vi "Drive Controller.vi"(8 "error in":errorcluster) -> ()   [LabVIEW 2017]
doc: "This VI executes continuously carrying out the current operation and responding to updates or new operation requests. It will often contain the timing or control code that is difficult to place directly in TeleOp. This VI generally opens all sensors and motors and isolates the rest of the robot code from knowing implementation details of how the operations are carried out."
uses:
  Drive Setpoints.ctl
  Drive Operations.ctl
  <vilib>/Rock Robotics/WPI/Solenoid/WPI_SolenoidChannel.ctl
  <vilib>/Rock Robotics/WPI/SafetyOutput/WPI_SafetyOutputConfigMenu.ctl
  Users/Public/Documents/Cross The Road Electronics/Phoenix-LabVIEW/Motor Controller/Controls/CTRE_Phoenix_MotorControl_ControlMode.ctl
  <vilib>/Rock Robotics/WPI/ThirdParty/Phoenix-LabVIEW/Motor Controller/Controls/CTRE_Phoenix_MotorControl_NeutralMode.ctl
  <vilib>/Rock Robotics/WPI/ThirdParty/Phoenix-LabVIEW/Motor Controller/Controls/CTRE_Phoenix_MotorControl_FeedbackDevice.ctl
  <vilib>/Rock Robotics/WPI/Solenoid/WPI_SolenoidValue.ctl
  <vilib>/Rock Robotics/WPI/ThirdParty/Phoenix-LabVIEW/Motor Controller/Controls/CTRE_Phoenix_MotorControl_StatusFrameEnhanced.ctl
  <vilib>/Rock Robotics/WPI/Solenoid/WPI_SolenoidOpenSingle.vi
  <vilib>/Rock Robotics/WPI/Solenoid/WPI_SolenoidSetEnum.vi
  <vilib>/Rock Robotics/WPI/Utilities/WPI_GetSetVariantRefNum.vi
  <vilib>/Rock Robotics/WPI/RobotDrive/WPI_RobotDriveMecanumDrive_Cartesian.vi
  <vilib>/Rock Robotics/WPI/ThirdParty/Phoenix-LabVIEW/Motor Controller/Get/CTRE_Phoenix_MotorController_GetQuadratureData.vi
panel:
  in  "P 2":dbl=0.8 format="%#_13g"
  in  "D":dbl format="%#_13g"
  in  "F 2":dbl=0.578
  in  "F":dbl=0.578
  out "Current\nCmd":string
  # ".578"
  # "Tip: It may be helpful to observe inputs and sensor values.\nYou may also want to display tuning or debugging controls."
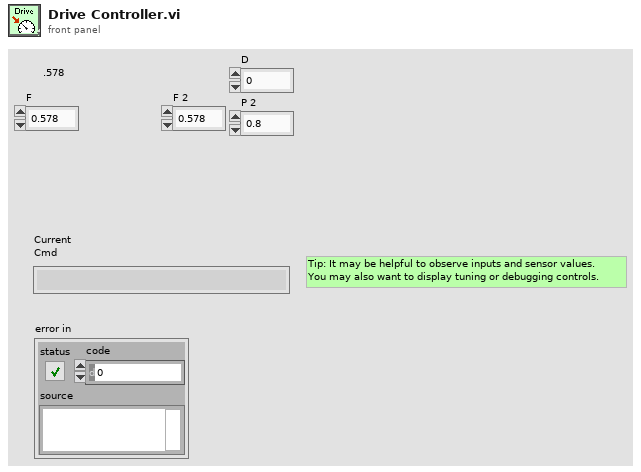
[diagram p1: front panel]
types:
  T1 = typedef "WPI_SolenoidChannel.ctl" = enum8{"Solenoid 0", "Solenoid 1", "Solenoid 2", "Solenoid 3", "Solenoid 4", "Solenoid 5", "Solenoid 6", "Solenoid 7", "Invalid"}
  T2 = typedef "CTRE_Phoenix_MotorControl_FeedbackDevice.ctl" = i8
  T3 = typedef "CTRE_Phoenix_MotorControl_NeutralMode.ctl" = enum8{"EEPROMSetting", "Override to Coast", "Override to Brake"}
  T4 = typedef "CTRE_Phoenix_MotorControl_ControlMode.ctl" = u16
  T5 = typedef "WPI_SafetyOutputConfigMenu.ctl" = enum16{"Enable", "Disable"}
  T6 = typedef "Drive Setpoints.ctl" = cluster{"Operation":T7, "X Setpoint":dbl, "Y Setpoint":dbl, "Duration":dbl, "Z Setpoint":dbl, "Tracks":bool, "Gyro":dbl, "POV":i16, "Distance(feet)":dbl, "AutoTrack Toggle":bool, "Collsision Detection":bool, "Reset Encoder":bool, "MP File Name":string}
  T7 = typedef "Drive Operations.ctl" = enum16{"Reserve", "Read Current", "Reset Motors VBus", "Motion Profile run", "Immediate Robot Centric", "Drive for Time Robot Centric", "Immediate Field Centric", "Drive For Time Field Centric", "Button Adjust", "Set Motors Motion Profile", "Reset Encoders", "Motion Profile Enable", "Drive for Distance"}
  T8 = typedef "WPI_MotorControlDeviceRef.ctl" = cluster{"DeviceStatus":errorcluster, "Type":T9, "PWM":cluster{"PWM Channel":T10, "DeadBand":T11}, "CAN":cluster{"Device Number":u8, "SetOutput VI Ref":variant, "GetOutput VI Ref":variant, "Enable VI Ref":variant, "Disable VI Ref":variant, "Data":variant}, "Invert":bool, "DIO PWM":cluster{"PWM \"Enable\" Channel":T10, "DIOChannel":T12, "PWM Rate":dbl}}
  T9 = typedef "WPI_MotorControlType.ctl" = enum16{"PWM", "CAN", "DIO PWM"}
  T10 = typedef "FPGA_DIOPWMChannel.ctl" = enum8{"PWM 0", "PWM 1", "PWM 2", "PWM 3", "PWM 4", "PWM 5", "PWM 6", "PWM 7", "PWM 8", "PWM 9", "PWM MXP 0", "PWM MXP 1", "PWM MXP 2", "PWM MXP 3", "PWM MXP 4", "PWM MXP 5", "PWM MXP 6", "PWM MXP 7", "PWM MXP 8", "PWM MXP 9", "Invalid"}
  T11 = typedef "WPI_PWMDeadband.ctl" = cluster{"Name":string, "maxPositivePwm":i32, "minPositivePwm":i32, "centerPwm":i32, "maxNegativePwm":i32, "minNegativePwm":i32, "angularRange":u16}
  T12 = typedef "FPGA_DIOChannel.ctl" = enum8{"DIO 0", "DIO 1", "DIO 2", "DIO 3", "DIO 4", "DIO 5", "DIO 6", "DIO 7", "DIO 8", "DIO 9", "DIO MXP 0", "DIO MXP 1", "DIO MXP 2", "DIO MXP 3", "DIO MXP 4", "DIO MXP 5", "DIO MXP 6", "DIO MXP 7", "DIO MXP 8", "DIO MXP 9", "DIO MXP 10", "DIO MXP 11", "DIO MXP 12", "DIO MXP 13", "DIO MXP 14", "DIO MXP 15", "SPI Port CS1", "SPI Port CS2", "SPI Port CS3", "SPI Port MISO", "SPI Port MOSI", "Invalid"}
  T13 = typedef "WPI_RobotDriveDevRef.ctl" = cluster{"DevStatus":errorcluster, "Motors[]":T8[], "Square Inputs":bool, "Max Output":dbl}
  T14 = typedef "WPI_SolenoidDevRef.ctl" = cluster{"DevStatus":errorcluster, "Pneumatics Control Module":u8, "Forward Solenoid Channel":T1, "Reverse Solenoid Channel":T1}
  T15 = typedef "Command Status Info.ctl" = cluster{"Name":string, "Status":T16, "notifier out":T17}
  T16 = typedef "Completion Status.ctl" = enum16{"Successful", "Aborted", "Incomplete"}
  T17 = typedef "Completion Notifier.ctl" = refnum<notifier>
  T18 = cluster{"SubSystem Data":T6, cluster{"Start Time (ms)":u32, "Iterations":i32}, cluster{"Command Info":T15, "Description":string, "SubSystem Data":T6, "notifier out":refnum<notifier>, "Subsystem Name":string}}
  T19 = typedef "WPI_SolenoidValue.ctl" = enum16{"Off", "On", "Forward", "Reverse"}
  T20 = typedef "CTRE_Phoenix_MotorControl_StatusFrameEnhanced.ctl" = u16
  T21 = cluster{"SubSystem Data":T6, cluster{"Start Time (ms)":u32, "Iterations":i32}, "Default Command Arguments":cluster{"Command Info":T15, "Description":string, "SubSystem Data":T6, "notifier out":refnum<notifier>, "Subsystem Name":string}}
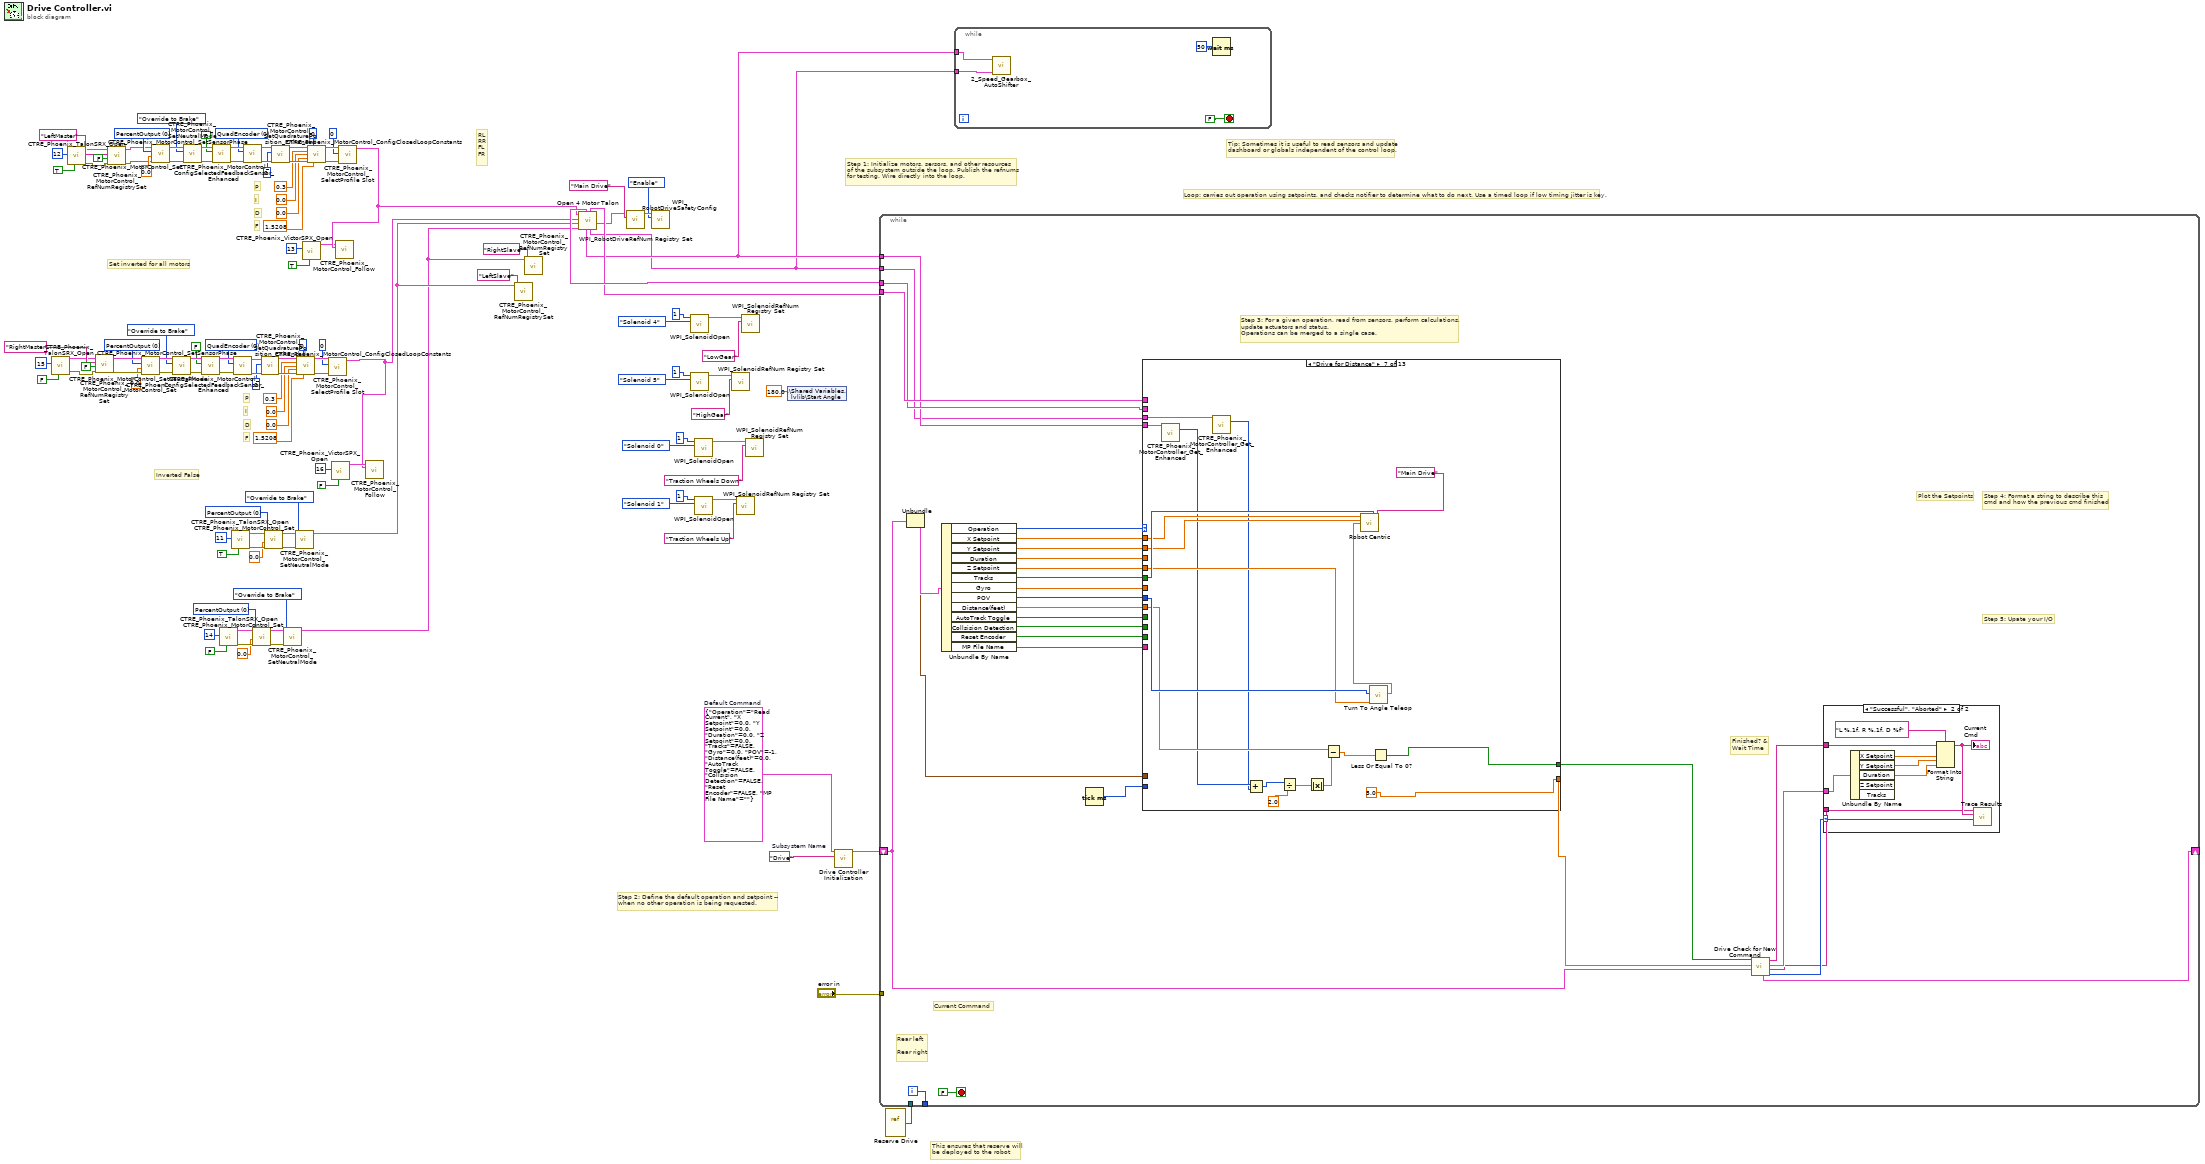
[diagram p0: block diagram]
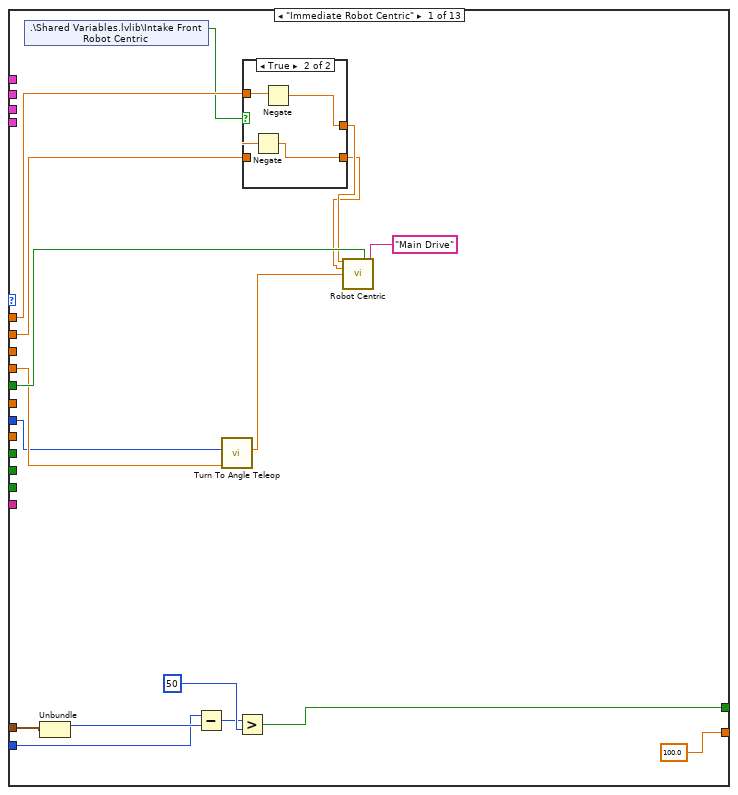
[diagram p3: hidden frame]
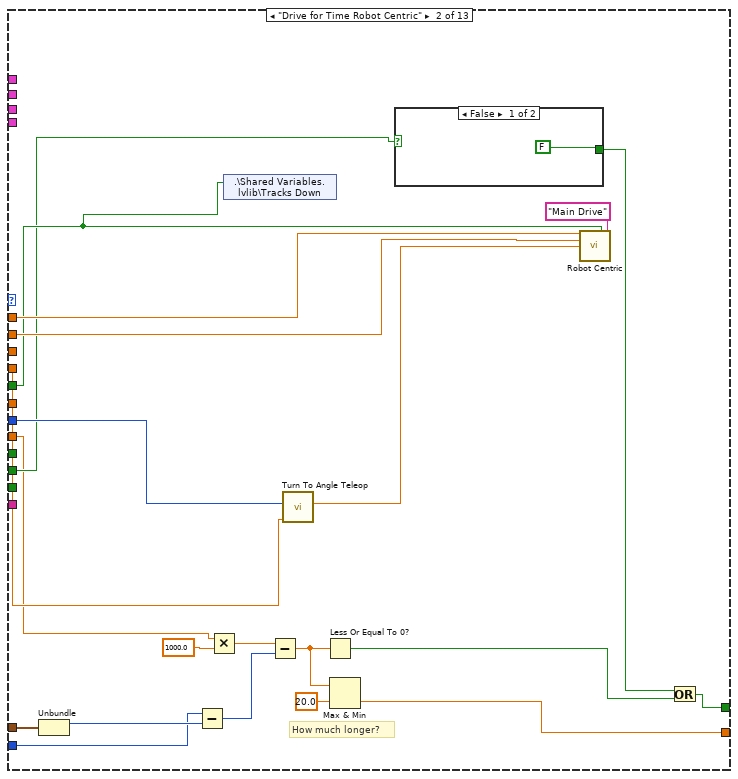
[diagram p5: hidden frame]
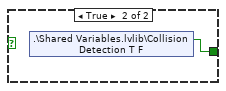
[diagram p6: hidden frame]
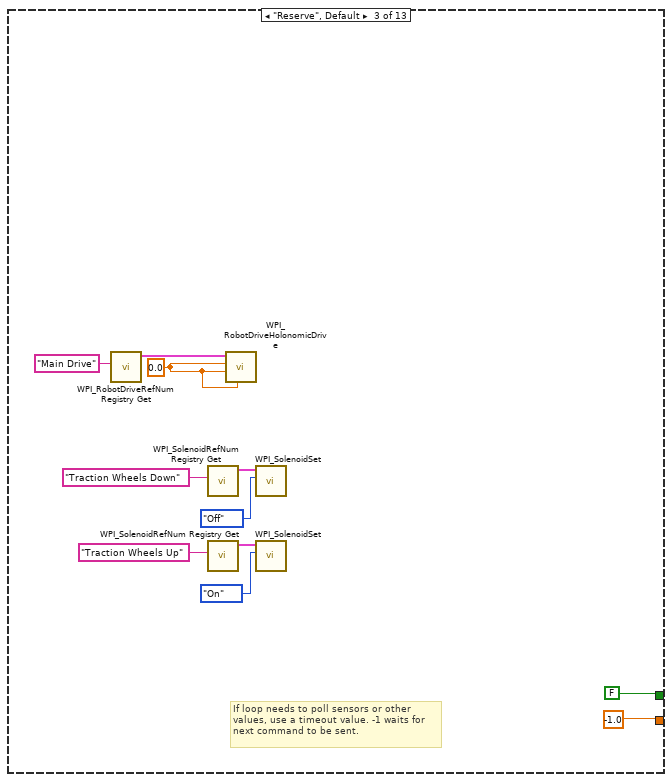
[diagram p7: hidden frame]
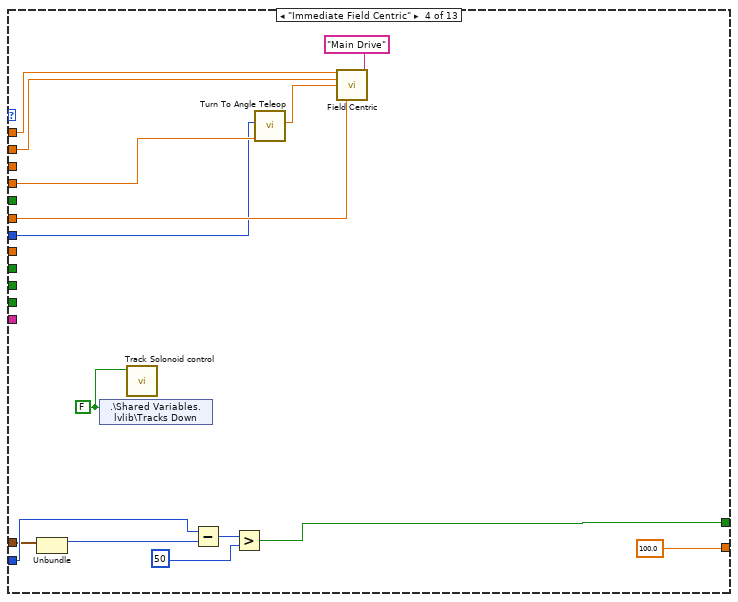
[diagram p8: hidden frame]
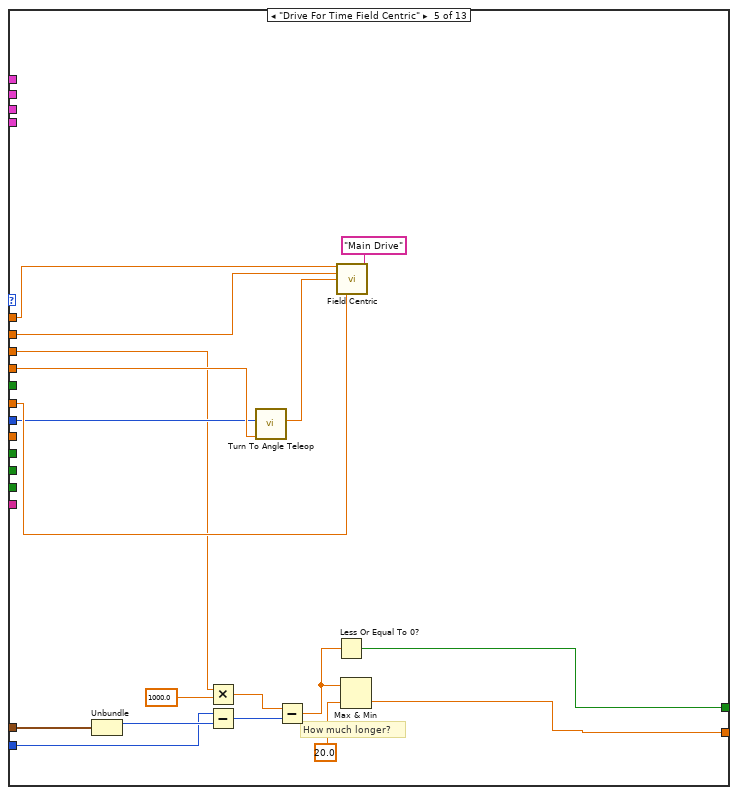
[diagram p9: hidden frame]
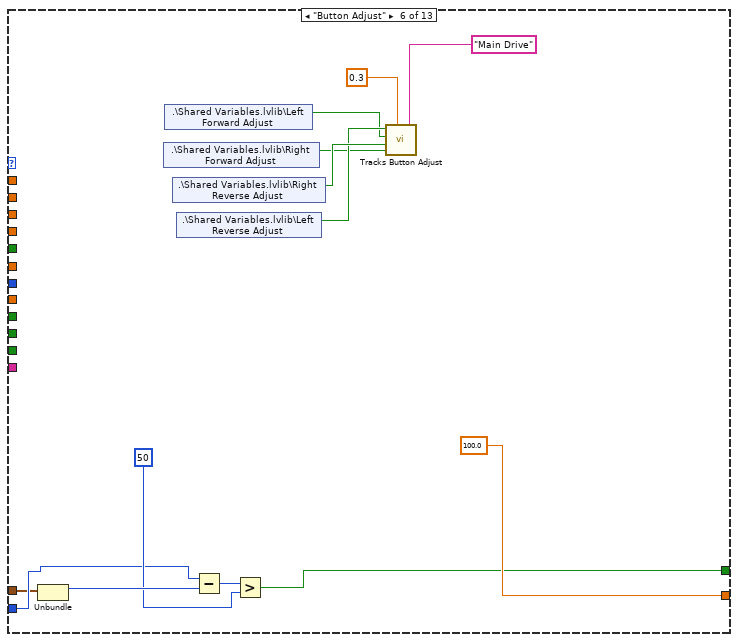
[diagram p10: hidden frame]
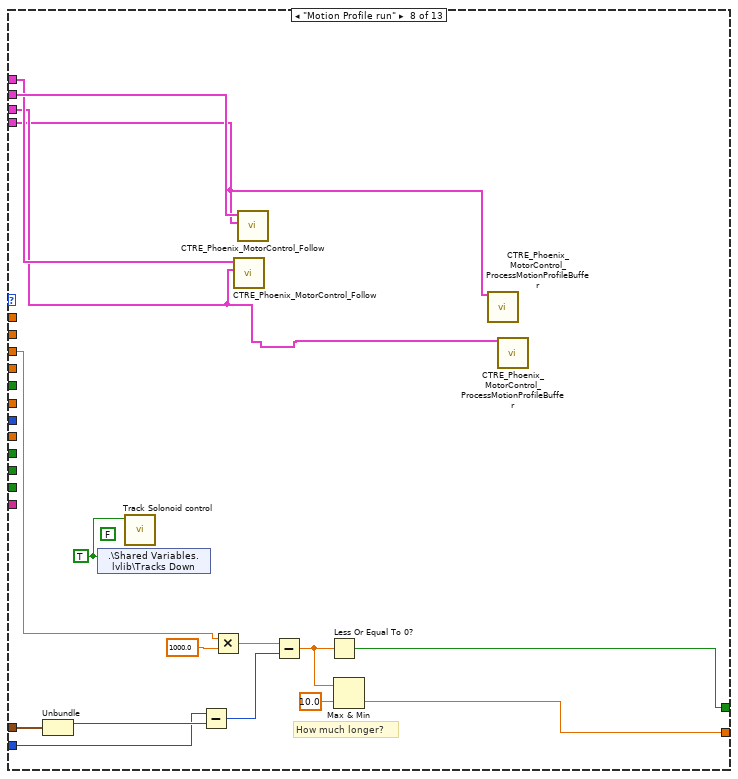
[diagram p11: hidden frame]
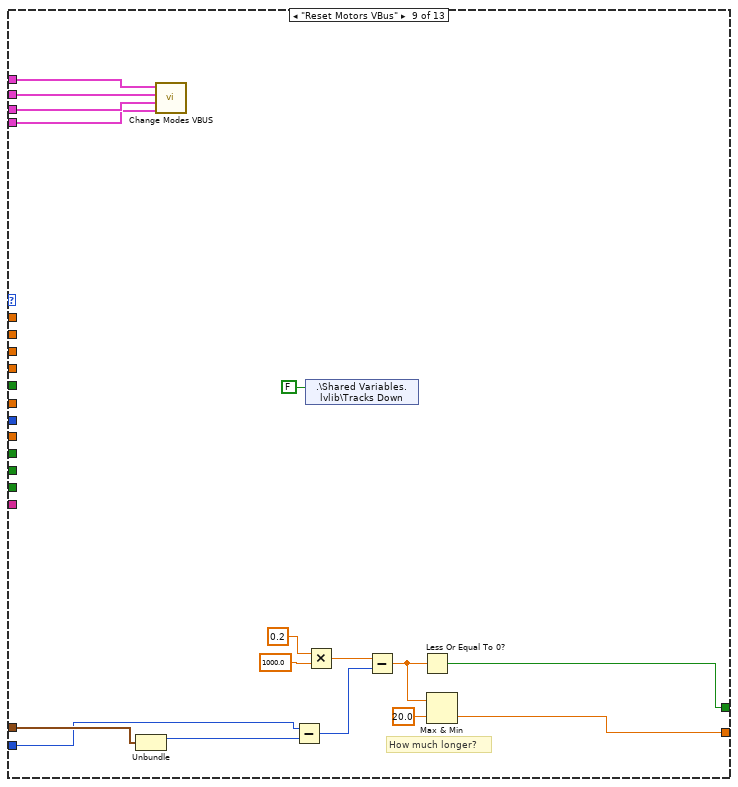
[diagram p12: hidden frame]
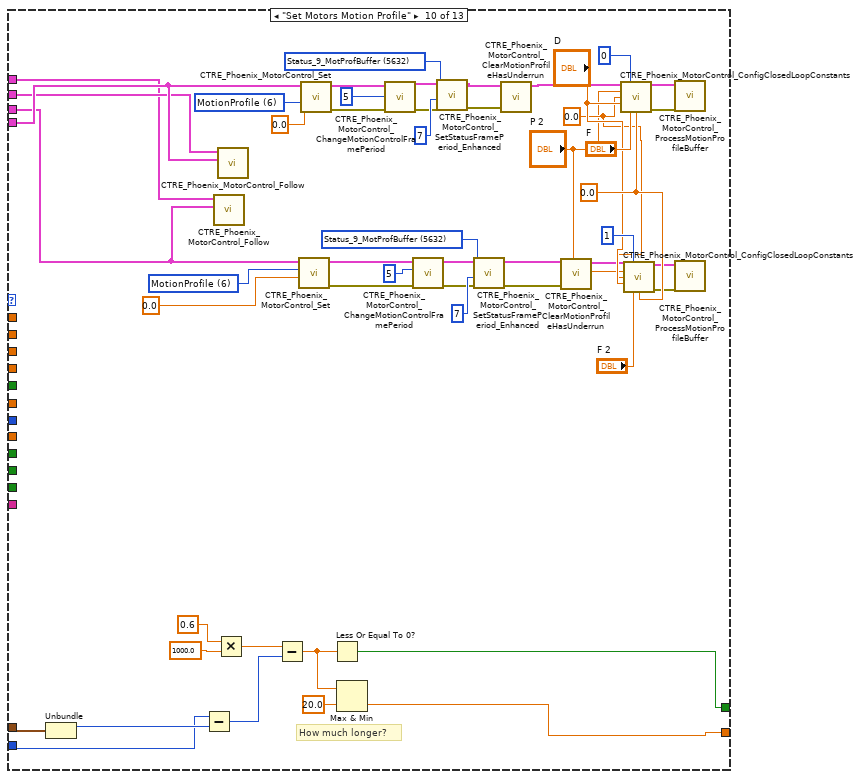
[diagram p13: hidden frame]
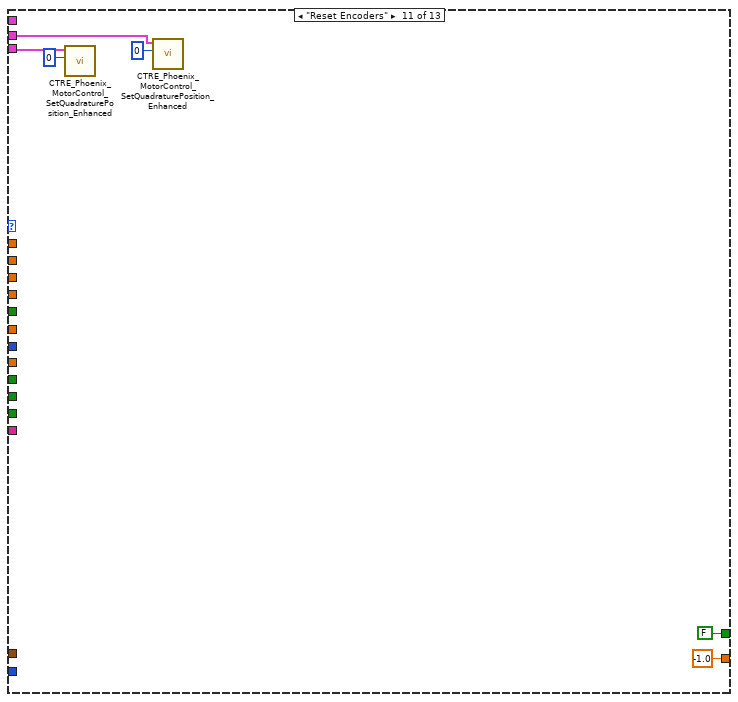
[diagram p14: hidden frame]
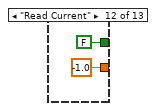
[diagram p15: hidden frame]
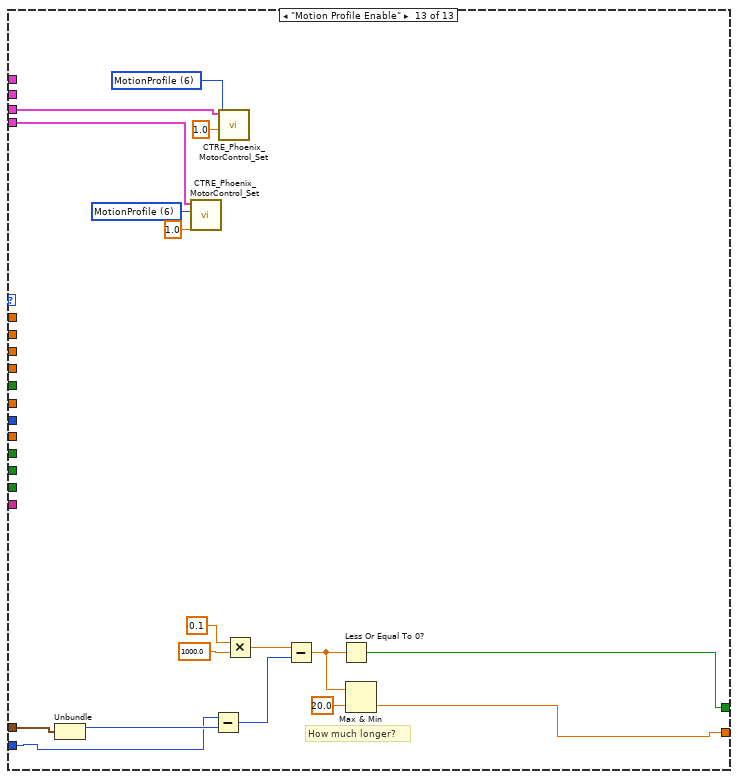
[diagram p16: hidden frame]
diagram:
  w32 = T2 0 items=["None"=-1, "QuadEncoder"=0, "Analog"=2, "Tachometer"=4, "Pulse Width Encoded Position"=8, "Sensor Sum (S0 + S1)"=9, "Sensor Difference (D0 - D1)"=10, "Remote Source 0"=11, "Remote Source 1"=12, "Software Emulated"=15] ("Feedback Device")
  w15 = T4 0 items=["PercentOutput"=0, "Position"=1, "Velocity"=2, "Current"=3, "Follower"=5, "MotionProfile"=6, "MotionMagic"=7, "MotionMagicArc"=8, "MotionProfileArc"=10, "Disabled"=15] ("Control Mode")
  w62 = T2 0 items=["None"=-1, "QuadEncoder"=0, "Analog"=2, "Tachometer"=4, "Pulse Width Encoded Position"=8, "Sensor Sum (S0 + S1)"=9, "Sensor Difference (D0 - D1)"=10, "Remote Source 0"=11, "Remote Source 1"=12, "Software Emulated"=15] ("Feedback Device")
  w47 = T4 0 items=["PercentOutput"=0, "Position"=1, "Velocity"=2, "Current"=3, "Follower"=5, "MotionProfile"=6, "MotionMagic"=7, "MotionMagicArc"=8, "MotionProfileArc"=10, "Disabled"=15] ("Control Mode")
  w78 = T4 0 items=["PercentOutput"=0, "Position"=1, "Velocity"=2, "Follower"=5, "MotionProfile"=6, "MotionMagic"=7, "MotionMagicArc"=8, "TimedPercentOutput"=9, "Disabled"=15] ("Control Mode")
  w86 = T4 0 items=["PercentOutput"=0, "Position"=1, "Velocity"=2, "Follower"=5, "MotionProfile"=6, "MotionMagic"=7, "MotionMagicArc"=8, "TimedPercentOutput"=9, "Disabled"=15] ("Control Mode")
  w123 = T6 {"Operation"=enum."Read Current", "X Setpoint"=0.0, "Y Setpoint"=0.0, "Duration"=0.0, "Z Setpoint"=0.0, "Tracks"=FALSE, "Gyro"=0.0, "POV"=-1, "Distance(feet)"=0.0, "AutoTrack Toggle"=FALSE, "Collsision Detection"=FALSE, "Reset Encoder"=FALSE, "MP File Name"=""}  # Default Command
  w124 = "Drive"  # Subsystem Name
  # "F"
  # "D"
  # "I"
  # "P"
  # "F"
  # "D"
  # "I"
  # "P"
  # "Set inverted for all motors"
  # "Inverted False"
  # "RL\nRR\nFL\nFR"
  # "This ensures that reserve will\nbe deployed to the robot"
  # "Tip: Sometimes it is useful to read sensors and update\ndashboard or globals independent of the control loop."
  # "Step 2: Define the default operation and setpoint --\nwhen no other operation is being requested."
  # "Step 1: Initialize motors, sersors, and other resources\nof the subsystem outside the loop. Publish the refnums\nfor testing. Wire directly into the loop."
  # "Loop: carries out operation using setpoints, and checks notifier to determine what to do next. Use a timed loop if low timing jitter is key."
  n1 = call <vilib>:"CTRE_Phoenix_TalonSRX_Open.vi"("Invert"=FALSE, "Device Number"=u8 15) -> ("error out"=w95:errorcluster, "CAN Talon SRX Ref"=w96:T8)  [unwired: 8 in]
  n2 = call <vilib>:"CTRE_Phoenix_TalonSRX_Open.vi"("Invert"=TRUE, "Device Number"=u8 12) -> ("error out"=w97:errorcluster, "CAN Talon SRX Ref"=w98:T8)  [unwired: 8 in]
  n3 = call <vilib>:"CTRE_Phoenix_MotorControl_RefNumRegistrySet.vi"("error in (no error)"=w95, "Test Mode Only"=FALSE, "refnum name"="RightMaster", "PhoenixMotorControlDevRef"=w96) -> ("error out"=w17:errorcluster, "PhoenixMotorControlDevRef"=w18:T8)  [unwired: 6 in]
  n4 = call <vilib>:"CTRE_Phoenix_MotorControl_RefNumRegistrySet.vi"("error in (no error)"=w97, "Test Mode Only"=FALSE, "refnum name"="LeftMaster", "PhoenixMotorControlDevRef"=w98) -> ("error out"=w45:errorcluster, "PhoenixMotorControlDevRef"=w46:T8)  [unwired: 6 in]
  n5 = call <vilib>:"CTRE_Phoenix_MotorControl_Set.vi"("error in (no error)"=w17, "Output"=0.0, "Control Mode"=w15, "PhoenixMotorControlDevRef"=w18) -> ("error out"=w36:errorcluster, "PhoenixMotorControlDevRef"=w40:T8)  [unwired: 6 in]
  n6 = call <vilib>:"CTRE_Phoenix_MotorControl_Set.vi"("error in (no error)"=w45, "Output"=0.0, "Control Mode"=w47, "PhoenixMotorControlDevRef"=w46) -> ("error out"=w66:errorcluster, "PhoenixMotorControlDevRef"=w70:T8)  [unwired: 6 in]
  n7 = call <vilib>:"CTRE_Phoenix_MotorControl_SetNeutralMode.vi"("error in (no error)"=w36, "Motor Control Neutral Mode"=CTRE_Phoenix_MotorControl_NeutralMode."Override to Brake", "PhoenixMotorControlDevRef"=w40) -> ("error out"=w38:errorcluster, "PhoenixMotorControlDevRef"=w37:T8)  [unwired: 7 in]
  n8 = call <vilib>:"CTRE_Phoenix_MotorControl_SetNeutralMode.vi"("error in (no error)"=w66, "Motor Control Neutral Mode"=CTRE_Phoenix_MotorControl_NeutralMode."Override to Brake", "PhoenixMotorControlDevRef"=w70) -> ("error out"=w68:errorcluster, "PhoenixMotorControlDevRef"=w67:T8)  [unwired: 7 in]
  n9 = call <vilib>:"CTRE_Phoenix_MotorControl_SetSensorPhase.vi"("error in (no error)"=w38, "PhaseSensor"=FALSE, "PhoenixMotorControlDevRef"=w37) -> ("error out"=w34:errorcluster, "PhoenixMotorControlDevRef"=w33:T8)  [unwired: 7 in]
  n10 = call <vilib>:"CTRE_Phoenix_MotorControl_SetSensorPhase.vi"("error in (no error)"=w68, "PhaseSensor"=FALSE, "PhoenixMotorControlDevRef"=w67) -> ("error out"=w64:errorcluster, "PhoenixMotorControlDevRef"=w63:T8)  [unwired: 7 in]
  n11 = call <vilib>:"CTRE_Phoenix_TalonSRX_Open.vi"("Invert"=FALSE, "Device Number"=u8 14) -> ("error out"=w80:errorcluster, "CAN Talon SRX Ref"=w79:T8)  [unwired: 8 in]
  n12 = call <vilib>:"CTRE_Phoenix_TalonSRX_Open.vi"("Invert"=TRUE, "Device Number"=u8 11) -> ("error out"=w88:errorcluster, "CAN Talon SRX Ref"=w87:T8)  [unwired: 8 in]
  n13 = call <vilib>:"CTRE_Phoenix_MotorControl_ConfigSelectedFeedbackSensor_Enhanced.vi"("error in (no error)"=w34, "Feedback Device"=w32, "PhoenixMotorControlDevRef"=w33) -> ("error out"=w30:errorcluster, "PhoenixMotorControlDevRef"=w31:T8)  [unwired: 7 in]
  n14 = call <vilib>:"CTRE_Phoenix_MotorControl_ConfigSelectedFeedbackSensor_Enhanced.vi"("error in (no error)"=w64, "Feedback Device"=w62, "PhoenixMotorControlDevRef"=w63) -> ("error out"=w60:errorcluster, "PhoenixMotorControlDevRef"=w61:T8)  [unwired: 7 in]
  n15 = call <vilib>:"CTRE_Phoenix_MotorControl_Set.vi"("error in (no error)"=w80, "Output"=0.0, "Control Mode"=w78, "PhoenixMotorControlDevRef"=w79) -> ("error out"=w75:errorcluster, "PhoenixMotorControlDevRef"=w74:T8)  [unwired: 6 in]
  n16 = call <vilib>:"CTRE_Phoenix_MotorControl_SetQuadraturePosition_Enhanced.vi"("error in (no error)"=w30, "New Position"=0, "PhoenixMotorControlDevRef"=w31) -> ("error out"=w27:errorcluster, "PhoenixMotorControlDevRef"=w28:T8)  [unwired: 7 in]
  n17 = call <vilib>:"CTRE_Phoenix_MotorControl_Set.vi"("error in (no error)"=w88, "Output"=0.0, "Control Mode"=w86, "PhoenixMotorControlDevRef"=w87) -> ("error out"=w83:errorcluster, "PhoenixMotorControlDevRef"=w82:T8)  [unwired: 6 in]
  n18 = call <vilib>:"CTRE_Phoenix_MotorControl_SetQuadraturePosition_Enhanced.vi"("error in (no error)"=w60, "New Position"=0, "PhoenixMotorControlDevRef"=w61) -> ("error out"=w57:errorcluster, "PhoenixMotorControlDevRef"=w58:T8)  [unwired: 7 in]
  n19 = call <vilib>:"CTRE_Phoenix_MotorControl_SetNeutralMode.vi"("error in (no error)"=w75, "Motor Control Neutral Mode"=CTRE_Phoenix_MotorControl_NeutralMode."Override to Brake", "PhoenixMotorControlDevRef"=w74) -> ("PhoenixMotorControlDevRef"=w9:T8)  [unwired: 7 in, 1 out]
  n20 = call <vilib>:"CTRE_Phoenix_MotorControl_SetNeutralMode.vi"("error in (no error)"=w83, "Motor Control Neutral Mode"=CTRE_Phoenix_MotorControl_NeutralMode."Override to Brake", "PhoenixMotorControlDevRef"=w82) -> ("PhoenixMotorControlDevRef"=w10:T8)  [unwired: 7 in, 1 out]
  n21 = call <vilib>:"CTRE_Phoenix_MotorControl_ConfigClosedLoopConstants.vi"("PhoenixMotorControlDevRef"=w28, "slotIdx"=0, "P"=0.3, "I"=0.0, "D"=0.0, "error in (no error)"=w27, "F"=1.5208) -> ("PhoenixMotorControlDevRef"=w20:T8, "error out"=w21:errorcluster)  [unwired: 7 in]
  n22 = call <vilib>:"CTRE_Phoenix_VictorSPX_Open.vi"("Invert"=TRUE, "Device Number"=u8 13) -> ("CAN Talon SRX Ref"=w43:T8)  [unwired: 8 in, 1 out]
  n23 = call <vilib>:"CTRE_Phoenix_MotorControl_ConfigClosedLoopConstants.vi"("PhoenixMotorControlDevRef"=w58, "slotIdx"=0, "P"=0.3, "I"=0.0, "D"=0.0, "error in (no error)"=w57, "F"=1.5208) -> ("PhoenixMotorControlDevRef"=w50:T8, "error out"=w51:errorcluster)  [unwired: 7 in]
  n24 = call <vilib>:"CTRE_Phoenix_MotorControl_SelectProfile Slot.vi"("error in (no error)"=w21, "slotIdx"=0, "PhoenixMotorControlDevRef"=w20) -> ("PhoenixMotorControlDevRef"=w13:T8)  [unwired: 7 in, 1 out]
  n25 = call <vilib>:"CTRE_Phoenix_VictorSPX_Open.vi"("Invert"=FALSE, "Device Number"=u8 16) -> ("CAN Talon SRX Ref"=w42:T8)  [unwired: 8 in, 1 out]
  n26 = call <vilib>:"CTRE_Phoenix_MotorControl_SelectProfile Slot.vi"("error in (no error)"=w51, "slotIdx"=0, "PhoenixMotorControlDevRef"=w50) -> ("PhoenixMotorControlDevRef"=w44:T8)  [unwired: 7 in, 1 out]
  n27 = call <vilib>:"CTRE_Phoenix_MotorControl_Follow.vi"("Master Controller to Follow"=w44, "PhoenixMotorControlDevRef"=w43) -> ()  [unwired: 8 in, 2 out]
  n28 = call <vilib>:"CTRE_Phoenix_MotorControl_Follow.vi"("Master Controller to Follow"=w13, "PhoenixMotorControlDevRef"=w42) -> ()  [unwired: 8 in, 2 out]
  n29 = call <vilib>:"CTRE_Phoenix_MotorControl_RefNumRegistrySet.vi"("refnum name"="LeftSlave", "PhoenixMotorControlDevRef"=w10) -> ()  [unwired: 8 in, 2 out]
  n30 = call <vilib>:"CTRE_Phoenix_MotorControl_RefNumRegistrySet.vi"("refnum name"="RightSlave", "PhoenixMotorControlDevRef"=w9) -> ()  [unwired: 8 in, 2 out]
  n31 = call "Open 4 Motor Talon.vi"("Front Right"=w9, "Front Left"=w10, "Rear Right"=w13, "Rear Left"=w44) -> ("RobotDriveDevRef"=w91:T13, "Rear Right"=w105:T8, "Front RIght"=w107:T8, "Rear Left"=w106:T8, "Front Left"=w108:T8)  [unwired: 3 in]
  n32 = call <vilib>:"WPI_RobotDriveRefNum Registry Set.vi"("refnum name"="Main Drive", "RobotDriveDevRef"=w91) -> ("RobotDriveDevRef"=w93:T13)  [unwired: 2 in, 7 out]
  n33 = call <vilib>:"WPI_RobotDriveSafetyConfig.vi"("mode"=WPI_SafetyOutputConfigMenu."Enable", "RobotDriveDevRef"=w93) -> ()  [unwired: 8 in, 2 out]
  n34 = call-poly <vilib>:"WPI_SolenoidOpen.vi"("Solenoid Channel"=WPI_SolenoidChannel."Solenoid 4", "Pneumatics Control Module (0)"=u8 1) -> ("SolenoidDevRef"=w4:T14)  [unwired: 8 in, 1 out]
  n35 = call-poly <vilib>:"WPI_SolenoidOpen.vi"("Solenoid Channel"=WPI_SolenoidChannel."Solenoid 5", "Pneumatics Control Module (0)"=u8 1) -> ("SolenoidDevRef"=w6:T14)  [unwired: 8 in, 1 out]
  n36 = call-poly <vilib>:"WPI_SolenoidOpen.vi"("Solenoid Channel"=WPI_SolenoidChannel."Solenoid 0", "Pneumatics Control Module (0)"=u8 1) -> ("SolenoidDevRef"=w113:T14)  [unwired: 8 in, 1 out]
  n37 = call-poly <vilib>:"WPI_SolenoidOpen.vi"("Solenoid Channel"=WPI_SolenoidChannel."Solenoid 1", "Pneumatics Control Module (0)"=u8 1) -> ("SolenoidDevRef"=w116:T14)  [unwired: 8 in, 1 out]
  n38 = call <vilib>:"WPI_SolenoidRefNum Registry Set.vi"("refnum name"="HighGear", "SolenoidDevRef"=w6) -> ()  [unwired: 8 in, 2 out]
  n39 = call <vilib>:"WPI_SolenoidRefNum Registry Set.vi"("refnum name"="Traction Wheels Up", "SolenoidDevRef"=w116) -> ()  [unwired: 8 in, 2 out]
  n40 = call <vilib>:"WPI_SolenoidRefNum Registry Set.vi"("refnum name"="LowGear", "SolenoidDevRef"=w4) -> ()  [unwired: 8 in, 2 out]
  n41 = call <vilib>:"WPI_SolenoidRefNum Registry Set.vi"("refnum name"="Traction Wheels Down", "SolenoidDevRef"=w113) -> ()  [unwired: 8 in, 2 out]
  n42 = shared-variable ".\\Shared Variables.lvlib\\Start Angle"(180.0 ("Start Angle")) -> ()  [unwired: 1 in, 1 out]
  n43 = call "Drive Controller Initialization.vi"("Subsystem Name"=w124, "Default Command"=w123) -> ("output cluster"=w121:T18)  [unwired: 9 in]
  n44 = vi-ref "Reserve Drive.vi"() -> (w120:refnum<vi>)
  n45 = while {
    shift-right: [w148] -> _
    shift-left: w121 -> [w137]
    tunnel: [w153] -> _
    tunnel: "error in" -> [_]
    tunnel: w120 -> [_]
    tunnel: w106 -> [w133]
    tunnel: w105 -> [w132]
    tunnel: w108 -> [w135]
    tunnel: w107 -> [w136]
    i -> [w153]
    stop <- FALSE stop-if-true
    # "Rear left \n\nRear right"
    # "Step 5: Upate your I/O"
    # "Step 4: Format a string to describe this\ncmd and how the previous cmd finished"
    # "Current Command"
    # "Plot the Setpoints"
    # "Finished? &\nWait Time"
    # "Step 3: For a given operation, read from sensors, perform calculations,\nupdate actuators and status.\nOperations can be merged to a single case."
    n46 = Unbundle(w137) -> ("SubSystem Data"=w152:T6, w144:cluster{"Start Time (ms)":u32, "Iterations":i32})  [unwired: 1 out]
    n47 = Unbundle By Name(w152) -> ("Operation"=w151:T7, "X Setpoint"=w140:dbl, "Y Setpoint"=w139:dbl, "Duration"=w130:dbl, "Z Setpoint"=w143:dbl, "Tracks"=w138:bool, "Gyro"=w142:dbl, "POV"=w131:i16, "Distance(feet)"=w129:dbl, "AutoTrack Toggle"=w128:bool, "Collsision Detection"=w127:bool, "Reset Encoder"=w125:bool, "MP File Name"=w126:string)
    n48 = Tick Count (ms)() -> (millisecond timer value=w150:u32)
    n49 = case shown="\"Drive for Distance\"" w151 {
      tunnel: [100.0 w200 -1.0 100.0 w244 100.0 5.0 ("y") w289 w302 w343 -1.0 ("y") -1.0 ("y") w378] -> w141
      tunnel: [w175 w194 FALSE ("ignore previous (F)") w229 w243 w261 w283 w288 w303 w342 FALSE ("ignore previous (F)") FALSE ("ignore previous (F)") w377] -> w134
      tunnel: w144 -> [w174 w205 _ w230 w246 w259 _ w293 w305 w345 _ _ w380]
      tunnel: w140 -> [w169 w197 _ w227 w241 _ w279 _ _ _ _ _ _]
      tunnel: w139 -> [w167 w196 _ w226 w253 _ w278 _ _ _ _ _ _]
      tunnel: w150 -> [w176 w203 _ w231 w245 w260 _ w292 w304 w344 _ _ w379]
      tunnel: w143 -> [w171 w190 _ w224 w238 _ w272 _ _ _ _ _ _]
      tunnel: w138 -> [w172 w192 _ _ _ _ w280 _ _ _ _ _ _]
      tunnel: w142 -> [_ _ _ w225 w240 _ _ _ _ _ _ _ _]
      tunnel: w131 -> [w165 w191 _ w222 w237 _ w274 _ _ _ _ _ _]
      tunnel: w126 -> [_ _ _ _ _ _ _ _ _ _ _ _ _]
      tunnel: w136 -> [_ _ _ _ _ _ _ w295 w317 w322 _ _ _]
      tunnel: w135 -> [_ _ _ _ _ _ _ w296 w316 w323 _ _ _]
      tunnel: w132 -> [_ _ _ _ _ _ w269 w287 w315 w324 w373 _ w393]
      tunnel: w133 -> [_ _ _ _ _ _ w270 w286 w314 w325 w374 _ w392]
      tunnel: w130 -> [_ _ _ _ w236 _ _ w291 _ _ _ _ _]
      tunnel: w129 -> [_ w187 _ _ _ _ w271 _ _ _ _ _ _]
      tunnel: w128 -> [_ _ _ _ _ _ _ _ _ _ _ _ _]
      tunnel: w127 -> [_ w188 _ _ _ _ _ _ _ _ _ _ _]
      tunnel: w125 -> [_ _ _ _ _ _ _ _ _ _ _ _ _]
      frame "Immediate Robot Centric" {
        n50 = shared-variable ".\\Shared Variables.lvlib\\Intake Front Robot Centric"() -> (w164:bool)  [unwired: 1 in, 1 out]
        n51 = Unbundle(w174) -> ("Start Time (ms)"=w177:u32)  [unwired: 1 out]
        n52 = Subtract(x=w176, y=w177) -> (x-y=w178:u32)
        n53 = call "Turn To Angle Teleop.vi"("Z Axis"=w171, "POV"=w165) -> ("Adjustment Voltage"=w170:dbl)  [unwired: 9 in]
        n54 = Greater?(x=w178, y=u8 50 ("Left Motor")) -> (0:w175:bool)
        n55 = case shown="True" w164 {
          tunnel: w169 -> [w182 w186]
          tunnel: [w182 w185] -> w168
          tunnel: w167 -> [w181 w184]
          tunnel: [w181 w183] -> w166
          frame False {
          }
          frame True {
            n56 = Negate(x=w184) -> (-x=w183:dbl)
            n57 = Negate(x=w186) -> (-x=w185:dbl)
          }
        }
        n58 = call "Robot Centric.vi"("X Axis"=w168, "Tracks Down"=w172, "Drive 1"="Main Drive", "Y Axis"=w166, "Z Axis"=w170) -> ()  [unwired: 11 in]
      }
      frame "Drive for Time Robot Centric" {
        # "How much longer?"
        n59 = Unbundle(w205) -> ("Start Time (ms)"=w204:u32)  [unwired: 1 out]
        n60 = Subtract(x=w203, y=w204) -> (x-y=w198:u32)
        n61 = Multiply(x=w187, y=1000.0) -> (x*y=w207:dbl)
        n62 = shared-variable ".\\Shared Variables.lvlib\\Tracks Down"(w192) -> ()  [unwired: 1 in, 1 out]
        n63 = Subtract(x=w207, y=w198) -> (x-y=w202:dbl)
        n64 = call "Turn To Angle Teleop.vi"("Z Axis"=w190, "POV"=w191) -> ("Adjustment Voltage"=w189:dbl)  [unwired: 9 in]
        n65 = Less Or Equal To 0?(x=w202) -> (x <= 0?=w195:bool)
        n66 = Max & Min(x=w202, y=20.0) -> (min(x,y)=w200:dbl)  [unwired: 1 out]
        n67 = case shown="False" w188 {
          tunnel: [FALSE w209] -> w193
          frame False {
          }
          frame True {
            n68 = shared-variable ".\\Shared Variables.lvlib\\Collision Detection T F"() -> (w209:bool)  [unwired: 1 in, 1 out]
          }
        }
        n69 = call "Robot Centric.vi"("X Axis"=w197, "Tracks Down"=w192, "Drive 1"="Main Drive", "Y Axis"=w196, "Z Axis"=w189) -> ()  [unwired: 11 in]
        n70 = Or(x=w193, y=w195) -> (x .or. y?=w194:bool)
      }
      frame "Reserve", Default {
        w216 = 0.0 ("X")
        # "If loop needs to poll sensors or other\nvalues, use a timeout value. -1 waits for\nnext command to be sent."
        n71 = call <vilib>:"WPI_RobotDriveRefNum Registry Get.vi"("refnum name"="Main Drive" ("Drive 1")) -> ("RobotDriveDevRef"=w218:T13)  [unwired: 9 in, 1 out]
        n72 = call <vilib>:"WPI_SolenoidRefNum Registry Get.vi"("refnum name"="Traction Wheels Down") -> ("SolenoidDevRef"=w213:T14)  [unwired: 9 in, 1 out]
        n73 = call <vilib>:"WPI_SolenoidRefNum Registry Get.vi"("refnum name"="Traction Wheels Up") -> ("SolenoidDevRef"=w212:T14)  [unwired: 9 in, 1 out]
        n74 = call-poly <vilib>:"WPI_RobotDriveHolonomicDrive.vi"("Rotation"=w216, "Y"=w216, "X"=w216, "RobotDriveDevRef"=w218) -> ()  [unwired: 5 in, 3 out]
        n75 = call-poly <vilib>:"WPI_SolenoidSet.vi"("Value"=WPI_SolenoidValue."Off", "SolenoidDevRef"=w213) -> ()  [unwired: 8 in, 2 out]
        n76 = call-poly <vilib>:"WPI_SolenoidSet.vi"("Value"=WPI_SolenoidValue."On", "SolenoidDevRef"=w212) -> ()  [unwired: 8 in, 2 out]
      }
      frame "Immediate Field Centric" {
        w221 = FALSE ("Tracks Down")
        n77 = Unbundle(w230) -> ("Start Time (ms)"=w232:u32)  [unwired: 1 out]
        n78 = shared-variable ".\\Shared Variables.lvlib\\Tracks Down"(w221) -> ()  [unwired: 1 in, 1 out]
        n79 = call "Track Solonoid control.vi"("Manual Tracks"=w221) -> ()  [unwired: 11 in]
        n80 = Subtract(x=w231, y=w232) -> (x-y=w233:u32)
        n81 = Greater?(x=w233, y=u8 50 ("Left Motor")) -> (0:w229:bool)
        n82 = call "Turn To Angle Teleop.vi"("Z Axis"=w224, "POV"=w222) -> ("Adjustment Voltage"=w223:dbl)  [unwired: 9 in]
        n83 = call "Field Centric.vi"("X Axis"=w227, "Drive 1"="Main Drive", "Y Axis"=w226, "Z Axis"=w223, "Gyro"=w225) -> ()  [unwired: 11 in]
      }
      frame "Drive For Time Field Centric" {
        # "How much longer?"
        n84 = Unbundle(w246) -> ("Start Time (ms)"=w249:u32)  [unwired: 1 out]
        n85 = Multiply(x=w236, y=1000.0) -> (x*y=w242:dbl)
        n86 = Subtract(x=w245, y=w249) -> (x-y=w251:u32)
        n87 = call "Turn To Angle Teleop.vi"("Z Axis"=w238, "POV"=w237) -> ("Adjustment Voltage"=w239:dbl)  [unwired: 9 in]
        n88 = Subtract(x=w242, y=w251) -> (x-y=w248:dbl)
        n89 = Less Or Equal To 0?(x=w248) -> (x <= 0?=w243:bool)
        n90 = call "Field Centric.vi"("X Axis"=w241, "Drive 1"="Main Drive", "Y Axis"=w253, "Z Axis"=w239, "Gyro"=w240) -> ()  [unwired: 11 in]
        n91 = Max & Min(x=w248, y=20.0) -> (min(x,y)=w244:dbl)  [unwired: 1 out]
      }
      frame "Button Adjust" {
        n92 = Unbundle(w259) -> ("Start Time (ms)"=w265:u32)  [unwired: 1 out]
        n93 = shared-variable ".\\Shared Variables.lvlib\\Right Forward Adjust"() -> (w255:bool)  [unwired: 1 in, 1 out]
        n94 = shared-variable ".\\Shared Variables.lvlib\\Left Forward Adjust"() -> (w254:bool)  [unwired: 1 in, 1 out]
        n95 = shared-variable ".\\Shared Variables.lvlib\\Right Reverse Adjust"() -> (w257:bool)  [unwired: 1 in, 1 out]
        n96 = shared-variable ".\\Shared Variables.lvlib\\Left Reverse Adjust"() -> (w256:bool)  [unwired: 1 in, 1 out]
        n97 = Subtract(x=w260, y=w265) -> (x-y=w264:u32)
        n98 = Greater?(x=w264, y=u8 50 ("Left Motor")) -> (0:w261:bool)
        n99 = call "Tracks Button Adjust.vi"("Left Forward Adjust"=w256, "Left Reverse Adjust"=w254, "Right Forward Adjust"=w257, "Right Reverse Adjust"=w255, "Adjust Speed"=0.3, "Drive 1"="Main Drive") -> ()  [unwired: 1 in]
      }
      frame "Drive for Distance" {
        n100 = call-poly <vilib>:"CTRE_Phoenix_MotorController_Get_Enhanced.vi"("PhoenixMotorControlDevRef"=w270) -> ("Quadrature Position"=w268:i32)  [unwired: 11 in, 3 out]
        n101 = call-poly <vilib>:"CTRE_Phoenix_MotorController_Get_Enhanced.vi"("PhoenixMotorControlDevRef"=w269) -> ("Quadrature Position"=w267:i32)  [unwired: 11 in, 3 out]
        n102 = Add(x=w268, y=w267) -> (x+y=w285:i32)
        n103 = Divide(x=w285, y=2.0) -> (x/y=w282:dbl)
        n104 = Absolute Value(x=w282) -> (abs(x)=w281:dbl)
        n105 = Subtract(x=w271, y=w281) -> (x-y=w276:dbl)
        n106 = call "Turn To Angle Teleop.vi"("Z Axis"=w272, "POV"=w274) -> ("Adjustment Voltage"=w273:dbl)  [unwired: 9 in]
        n107 = call "Robot Centric.vi"("X Axis"=w279, "Tracks Down"=w280, "Drive 1"="Main Drive", "Y Axis"=w278, "Z Axis"=w273) -> ()  [unwired: 11 in]
        n108 = Less Or Equal To 0?(x=w276) -> (x <= 0?=w283:bool)
      }
      frame "Motion Profile run" {
        (unwired) FALSE ("AutoTrack")
        w294 = TRUE ("Tracks Down")
        # "How much longer?"
        n109 = Unbundle(w293) -> ("Start Time (ms)"=w300:u32)  [unwired: 1 out]
        n110 = shared-variable ".\\Shared Variables.lvlib\\Tracks Down"(w294) -> ()  [unwired: 1 in, 1 out]
        n111 = call "Track Solonoid control.vi"("Manual Tracks"=w294) -> ()  [unwired: 11 in]
        n112 = Subtract(x=w292, y=w300) -> (x-y=w297:u32)
        n113 = Multiply(x=w291, y=1000.0) -> (x*y=w290:dbl)
        n114 = call <vilib>:"CTRE_Phoenix_MotorControl_Follow.vi"("Master Controller to Follow"=w287, "PhoenixMotorControlDevRef"=w295) -> ()  [unwired: 8 in, 2 out]
        n115 = call <vilib>:"CTRE_Phoenix_MotorControl_Follow.vi"("Master Controller to Follow"=w286, "PhoenixMotorControlDevRef"=w296) -> ()  [unwired: 8 in, 2 out]
        n116 = Subtract(x=w290, y=w297) -> (x-y=w299:dbl)
        n117 = Less Or Equal To 0?(x=w299) -> (x <= 0?=w288:bool)
        n118 = Max & Min(x=w299, y=10.0) -> (min(x,y)=w289:dbl)  [unwired: 1 out]
        n119 = call <vilib>:"CTRE_Phoenix_MotorControl_ProcessMotionProfileBuffer.vi"("PhoenixMotorControlDevRef"=w286) -> ()  [unwired: 13 in, 2 out]
        n120 = call <vilib>:"CTRE_Phoenix_MotorControl_ProcessMotionProfileBuffer.vi"("PhoenixMotorControlDevRef"=w287) -> ()  [unwired: 13 in, 2 out]
      }
      frame "Reset Motors VBus" {
        # "How much longer?"
        n121 = Unbundle(w305) -> ("Start Time (ms)"=w310:u32)  [unwired: 1 out]
        n122 = call "Change Modes VBUS.vi"("PhoenixMotorControlDevRef 4"=w314, "PhoenixMotorControlDevRef 3"=w315, "PhoenixMotorControlDevRef 2"=w316, "PhoenixMotorControlDevRef"=w317) -> ()  [unwired: 8 in]
        n123 = Subtract(x=w304, y=w310) -> (x-y=w307:u32)
        n124 = shared-variable ".\\Shared Variables.lvlib\\Tracks Down"(FALSE ("Tracks Down")) -> ()  [unwired: 1 in, 1 out]
        n125 = Multiply(x=0.2, y=1000.0) -> (x*y=w312:dbl)
        n126 = Subtract(x=w312, y=w307) -> (x-y=w309:dbl)
        n127 = Less Or Equal To 0?(x=w309) -> (x <= 0?=w303:bool)
        n128 = Max & Min(x=w309, y=20.0) -> (min(x,y)=w302:dbl)  [unwired: 1 out]
      }
      frame "Set Motors Motion Profile" {
        w336 = T20 5632 items=["Status_1_General"=5120, "Status_2_Feedback0"=5184, "Status_3_Quadrature"=5248, "Status_4_AinTempVbat"=5312, "Status_6_Misc"=5440, "Status_7_CommStatus"=5504, "Status_8_PulseWidth"=5568, "Status_9_MotProfBuffer"=5632, "Status_10_MotionMagic"=5696, "Status_11_UartGadgeteer"=5760, "Status_12_Feedback1"=5824, "Status_13_Base_PIDF0"=5888, "Status_14_Turn_PIDF1"=5952, "Status_15_FirmwareApiStatus"=6016] ("Status Frame")
        w338 = T20 5632 items=["Status_1_General"=5120, "Status_2_Feedback0"=5184, "Status_3_Quadrature"=5248, "Status_4_AinTempVbat"=5312, "Status_6_Misc"=5440, "Status_7_CommStatus"=5504, "Status_8_PulseWidth"=5568, "Status_9_MotProfBuffer"=5632, "Status_10_MotionMagic"=5696, "Status_11_UartGadgeteer"=5760, "Status_12_Feedback1"=5824, "Status_13_Base_PIDF0"=5888, "Status_14_Turn_PIDF1"=5952, "Status_15_FirmwareApiStatus"=6016] ("Status Frame")
        w356 = 0.0 ("P")
        w353 = 0.0 ("P")
        w363 = T4 6 items=["PercentOutput"=0, "Position"=1, "Velocity"=2, "Follower"=5, "MotionProfile"=6, "MotionMagic"=7, "MotionMagicArc"=8, "TimedPercentOutput"=9, "Disabled"=15] ("Control Mode")
        w368 = T4 6 items=["PercentOutput"=0, "Position"=1, "Velocity"=2, "Follower"=5, "MotionProfile"=6, "MotionMagic"=7, "MotionMagicArc"=8, "TimedPercentOutput"=9, "Disabled"=15] ("Control Mode")
        # "How much longer?"
        n129 = Unbundle(w345) -> ("Start Time (ms)"=w349:u32)  [unwired: 1 out]
        n130 = Subtract(x=w344, y=w349) -> (x-y=w346:u32)
        n131 = call <vilib>:"CTRE_Phoenix_MotorControl_Follow.vi"("Master Controller to Follow"=w324, "PhoenixMotorControlDevRef"=w322) -> ()  [unwired: 8 in, 2 out]
        n132 = Multiply(x=0.6, y=1000.0) -> (x*y=w351:dbl)
        n133 = call <vilib>:"CTRE_Phoenix_MotorControl_Follow.vi"("Master Controller to Follow"=w325, "PhoenixMotorControlDevRef"=w323) -> ()  [unwired: 8 in, 2 out]
        n134 = Subtract(x=w351, y=w346) -> (x-y=w348:dbl)
        n135 = call <vilib>:"CTRE_Phoenix_MotorControl_Set.vi"("Output"=0.0, "Control Mode"=w363, "PhoenixMotorControlDevRef"=w324) -> ("error out"=w359:errorcluster, "PhoenixMotorControlDevRef"=w361:T8)  [unwired: 7 in]
        n136 = call <vilib>:"CTRE_Phoenix_MotorControl_Set.vi"("Output"=0.0, "Control Mode"=w368, "PhoenixMotorControlDevRef"=w325) -> ("error out"=w364:errorcluster, "PhoenixMotorControlDevRef"=w365:T8)  [unwired: 7 in]
        n137 = Less Or Equal To 0?(x=w348) -> (x <= 0?=w342:bool)
        n138 = Max & Min(x=w348, y=20.0) -> (min(x,y)=w343:dbl)  [unwired: 1 out]
        n139 = call <vilib>:"CTRE_Phoenix_MotorControl_ChangeMotionControlFramePeriod.vi"("error in"=w364, "periodMs"=5, "PhoenixMotorControlDevRef"=w365) -> ("error out"=w329:errorcluster, "PhoenixMotorControlDevRef"=w335:T8)  [unwired: 7 in]
        n140 = call <vilib>:"CTRE_Phoenix_MotorControl_ChangeMotionControlFramePeriod.vi"("error in"=w359, "periodMs"=5, "PhoenixMotorControlDevRef"=w361) -> ("error out"=w327:errorcluster, "PhoenixMotorControlDevRef"=w340:T8)  [unwired: 7 in]
        n141 = call <vilib>:"CTRE_Phoenix_MotorControl_SetStatusFramePeriod_Enhanced.vi"("error in (no error)"=w329, "periodMs"=7, "Status Frame"=w336, "PhoenixMotorControlDevRef"=w335) -> ("error out"=w328:errorcluster, "PhoenixMotorControlDevRef"=w332:T8)  [unwired: 6 in]
        n142 = call <vilib>:"CTRE_Phoenix_MotorControl_SetStatusFramePeriod_Enhanced.vi"("error in (no error)"=w327, "periodMs"=7, "Status Frame"=w338, "PhoenixMotorControlDevRef"=w340) -> ("error out"=w326:errorcluster, "PhoenixMotorControlDevRef"=w334:T8)  [unwired: 6 in]
        n143 = call <vilib>:"CTRE_Phoenix_MotorControl_ClearMotionProfileHasUnderrun.vi"("error in"=w328, "PhoenixMotorControlDevRef"=w332) -> ("PhoenixMotorControlDevRef"=w331:T8)  [unwired: 8 in, 1 out]
        n144 = call <vilib>:"CTRE_Phoenix_MotorControl_ClearMotionProfileHasUnderrun.vi"("error in"=w326, "PhoenixMotorControlDevRef"=w334) -> ("PhoenixMotorControlDevRef"=w333:T8)  [unwired: 8 in, 1 out]
        n145 = call <vilib>:"CTRE_Phoenix_MotorControl_ConfigClosedLoopConstants.vi"("PhoenixMotorControlDevRef"=w331, "slotIdx"=0, "P"="P 2", "I"=w353, "D"="D", "F"="F", "I Zone"=w356) -> ("PhoenixMotorControlDevRef"=w321:T8, "error out"=w320:errorcluster)  [unwired: 7 in]
        n146 = call <vilib>:"CTRE_Phoenix_MotorControl_ConfigClosedLoopConstants.vi"("PhoenixMotorControlDevRef"=w333, "slotIdx"=1, "P"="P 2", "I"=w353, "D"="D", "F"="F 2", "I Zone"=w356) -> ("PhoenixMotorControlDevRef"=w319:T8, "error out"=w318:errorcluster)  [unwired: 7 in]
        n147 = call <vilib>:"CTRE_Phoenix_MotorControl_ProcessMotionProfileBuffer.vi"("PhoenixMotorControlDevRef"=w321, "error in"=w320) -> ()  [unwired: 12 in, 2 out]
        n148 = call <vilib>:"CTRE_Phoenix_MotorControl_ProcessMotionProfileBuffer.vi"("PhoenixMotorControlDevRef"=w319, "error in"=w318) -> ()  [unwired: 12 in, 2 out]
      }
      frame "Reset Encoders" {
        n149 = call <vilib>:"CTRE_Phoenix_MotorControl_SetQuadraturePosition_Enhanced.vi"("New Position"=0, "PhoenixMotorControlDevRef"=w374) -> ()  [unwired: 8 in, 2 out]
        n150 = call <vilib>:"CTRE_Phoenix_MotorControl_SetQuadraturePosition_Enhanced.vi"("New Position"=0, "PhoenixMotorControlDevRef"=w373) -> ()  [unwired: 8 in, 2 out]
      }
      frame "Read Current" {
      }
      frame "Motion Profile Enable" {
        w388 = T4 6 items=["PercentOutput"=0, "Position"=1, "Velocity"=2, "Current"=3, "Follower"=5, "MotionProfile"=6, "MotionMagic"=7, "MotionMagicArc"=8, "MotionProfileArc"=10, "Disabled"=15] ("Control Mode")
        w391 = T4 6 items=["PercentOutput"=0, "Position"=1, "Velocity"=2, "Current"=3, "Follower"=5, "MotionProfile"=6, "MotionMagic"=7, "MotionMagicArc"=8, "MotionProfileArc"=10, "Disabled"=15] ("Control Mode")
        # "How much longer?"
        n151 = Unbundle(w380) -> ("Start Time (ms)"=w385:u32)  [unwired: 1 out]
        n152 = call <vilib>:"CTRE_Phoenix_MotorControl_Set.vi"("Output"=1.0, "Control Mode"=w391, "PhoenixMotorControlDevRef"=w392) -> ()  [unwired: 7 in, 2 out]
        n153 = Subtract(x=w379, y=w385) -> (x-y=w382:u32)
        n154 = call <vilib>:"CTRE_Phoenix_MotorControl_Set.vi"("Output"=1.0, "Control Mode"=w388, "PhoenixMotorControlDevRef"=w393) -> ()  [unwired: 7 in, 2 out]
        n155 = Multiply(x=0.1, y=1000.0) -> (x*y=w387:dbl)
        n156 = Subtract(x=w387, y=w382) -> (x-y=w384:dbl)
        n157 = Less Or Equal To 0?(x=w384) -> (x <= 0?=w377:bool)
        n158 = Max & Min(x=w384, y=20.0) -> (min(x,y)=w378:dbl)  [unwired: 1 out]
      }
    }
    n159 = call "Drive Check for New Command.vi"("input cluster"=w137, "Wait time (ms)"=w141, "Finished?"=w134) -> ("Completion"=w149:T16, "Subsystem Name"=w145:string, "SetPoint"=w146:T6, "Initial Trace String"=w147:string, "output cluster"=w148:T21)  [unwired: 4 in]
    n160 = case shown="\"Successful\", \"Aborted\"" w149 {
      selector: w149 -> [_ w163]
      tunnel: w147 -> [_ w158]
      tunnel: w146 -> [_ w159]
      tunnel: w145 -> [_ w155]
      frame "Incomplete", Default {
        # "Continuing current command"
      }
      frame "Successful", "Aborted" {
        # "Report and setup for next command"
        n161 = Unbundle By Name(w159) -> ("X Setpoint"=w161:dbl, "Y Setpoint"=w162:dbl, "Duration"=w156:dbl)  [unwired: 2 out]
        n162 = Format Into String(format string="L %.1f, R %.1f, D %f", initial string=w158, w161, w162, w156) -> (resulting string=w157:string)  [unwired: 1 in, 1 out]
        "Current\nCmd" <- w157
        n163 = call <vilib>:"Trace Results.vi"("Status of previous command"=w163, "Description"=w157, "Subsystem"=w155) -> ()  [unwired: 9 in]
      }
    }
  }
  n164 = while {
    tunnel: w106 -> [w394]
    tunnel: w105 -> [w395]
    stop <- FALSE stop-if-true
    n165 = call "2_Speed_Gearbox_AutoShifter.vi"("PhoenixMotorControlDevRef 2"=w395, "PhoenixMotorControlDevRef"=w394) -> ()  [unwired: 10 in]
    n166 = Wait (ms)(milliseconds to wait=u32 50) -> ()  [unwired: 1 out]
  }
